vi "NovaTech409A_WriteAndRead.vi"(3 "error in (no error)":errorcluster, 4 "Number of Bytes":i32=-1, 5 "write buffer":string="R\n", 6 "VISA resource name":refnum<visa-resource-name>="COM1") -> (0 "error out":errorcluster, 1 "read buffer":string, 2 "VISA resource name out":refnum<visa-resource-name>="COM1")   [LabVIEW 2013, in "Novatech 409A.lvlib"]
uses:
  Novatech 409A.lvlib
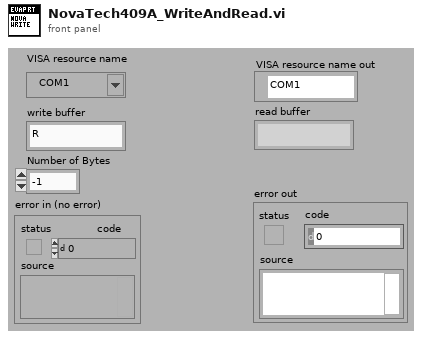
[diagram p1: front panel]
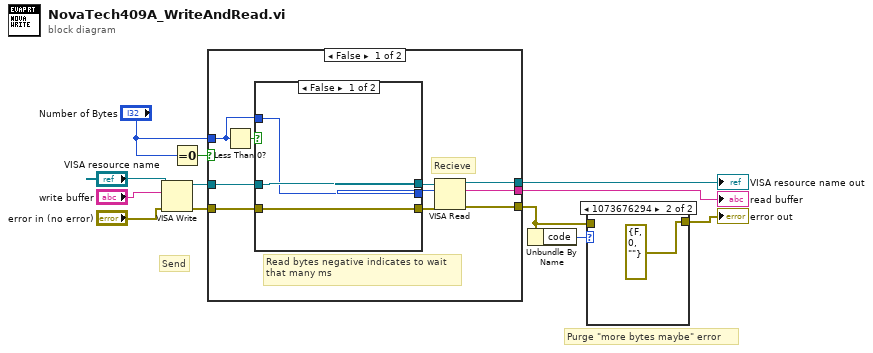
[diagram p0: block diagram]
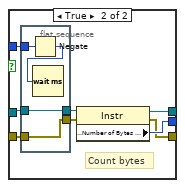
[diagram p2: hidden frame]
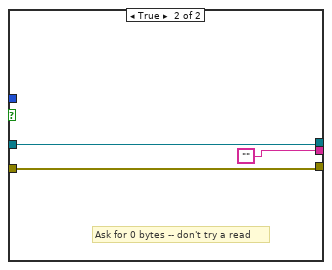
[diagram p3: hidden frame]
diagram:
  # "Purge \"more bytes maybe\" error"
  # "Send"
  n1 = VISA Write(VISA resource name="VISA resource name", write buffer="write buffer", error in (no error)="error in (no error)") -> (VISA resource name out=w7:refnum<visa-resource-name>, error out=w6:errorcluster)  [unwired: 1 out]
  n2 = Equal To 0?(x="Number of Bytes") -> (x = 0?=w2:bool)
  n3 = case shown="False" w2 {
    tunnel: [w22 ""] -> w12
    tunnel: [w21 w40] -> w8
    tunnel: w7 -> [w19 w40]
    tunnel: w6 -> [w18 w39]
    tunnel: [w15 w39] -> w4
    tunnel: "Number of Bytes" -> [w13 _]
    frame False {
      # "Read bytes negative indicates to wait\nthat many ms"
      # "Recieve"
      n4 = Less Than 0?(x=w13) -> (x < 0?=w14:bool)
      n5 = case shown="False" w14 {
        tunnel: [w23 w32] -> w20
        tunnel: w19 -> [w24 w29]
        tunnel: w18 -> [w25 w28]
        tunnel: [w25 w31] -> w17
        tunnel: [w24 w33] -> w16
        tunnel: w13 -> [w23 w26]
        frame False {
        }
        frame True {
          # "Count bytes"
          n6 = flat-sequence {
            tunnel: [w37] -> w30
            tunnel: w29 -> [w37]
            tunnel: w28 -> [w36]
            tunnel: [w36] -> w27
            tunnel: w26 -> [w35]
            frame #0 {
              n7 = Negate(x=w35) -> (-x=w34:i32)
              n8 = Wait (ms)(milliseconds to wait=w34) -> ()  [unwired: 1 out]
            }
          }
          n9 = property class="Instr"(reference=w30, error in=w27) -> (reference out=w33:refnum<visa-resource-name>, error out=w31:errorcluster, "Serial Settings:Number of Bytes at Serial Port"=w32:u32)
        }
      }
      n10 = VISA Read(VISA resource name=w16, byte count=w20, error in (no error)=w17) -> (VISA resource name out=w21:refnum<visa-resource-name>, read buffer=w22:string, error out=w15:errorcluster)  [unwired: 1 out]
    }
    frame True {
      # "Ask for 0 bytes -- don't try a read"
    }
  }
  "read buffer" <- w12
  "VISA resource name out" <- w8
  n11 = Unbundle By Name(w4) -> ("code"=w5:i32)
  n12 = case shown="1073676294" w5 {
    tunnel: w4 -> [w41 _]
    tunnel: [w41 errorcluster {"status"=FALSE, "code"=0, "source"=""} ("error in (no error)")] -> w3
    frame 0, Default {
    }
    frame 1073676294 {
    }
  }
  "error out" <- w3
